vi "Gui_SetupTimingScript.vi"(7 "Variant For Path":variant, 8 "error in (no error)":errorcluster, 11 "Variant":variant) -> (0 "error out":errorcluster caption="sortie d'erreur", 3 "Variant Output":variant)   [LabVIEW 2018]
uses:
  controls/EXPERT_Inputs.ctl
  controls/DIGIT_5122_Inputs.ctl
  <instrlib>/niScope/Controls/niScope trigger source.ctl
  controls/HSDIO_6541_Inputs.ctl
  <instrlib>/niHSDIO/niHSDIO.llb/niHSDIO_ctl Trigger Source Values (Ring).ctl
  controls/SOFTWARE_Inputs.ctl
  controls/AO_6711_Inputs.ctl
  controls/AWG_5421_Inputs.ctl
  <instrlib>/niFgen/niFgen.llb/niFgen_ctl Trigger Source Values (Ring).ctl
  controls/XML_Inputs.ctl
  controls/SEQUENCE_Inputs.ctl
  controls/EXCIT_Inputs.ctl
  controls/DATA_Inputs.ctl
  controls/TIMING_Inputs.ctl
  controls/PROCESSING_Inputs.ctl
  controls/TRAPPING_Inputs.ctl
panel:
  in  "SEQUENCE Inputs":T1={"EXCIT Inputs"={"Number of Excitations"=1, "Script Text"="", "Table of Waveforms"=[]}, "DATA Inputs"={"Record Length"=524000, "Sample Rate"=2000000.0, "Data Type"=0, "Vertical Range"=10.0, "Acquisition Duration"=262.0}, "TIMING Inputs"={"Number of Acquisitions "=1, "Number of Accumulations"=1, "Table of Waveforms"=[], "Script Text"=""}, "PROCESSING Inputs"={"Reference Mass"=300.0939, "Cyclotron Freq"=255.727, "Magnetron Freq"=0.001}, "TRAPPING Inputs"={"Number of Channels"=4, "Init Values"=[2.0, 9.0, 2.0, 9.0], "Opening Values"=[0.0, 0.0, 0.0, 0.0], "Trapping Values"=[2.0, 9.0, 2.0, 9.0], "Emptying Values"=[-10.0, -10.0, -10.0, -10.0], "Adiabatic ON"=FALSE, "Adiabatic Duration"=100, "Adiabatic Waveforms"=["Adiabatic_None_2_2_2000", "Adiabatic_Ramp_9_0_2000", "Adiabatic_None_2_2_2000", "Adiabatic_RC_9_0_2000"], "Ions Refill ON"=FALSE, "Number of Ions Refills"=1, "Trapping Delay"=400.0, "Trapping Duration"=300.0}} {"TRAPPING Inputs"."Trapping Duration" min=2.0; "TRAPPING Inputs"."Trapping Delay" min=2.0; "TRAPPING Inputs"."Number of Ions Refills" min=1 max=1000; "TRAPPING Inputs"."Trapping Values" min=-10.0 max=10.0; "TRAPPING Inputs"."Init Values" min=-10.0 max=10.0; "TRAPPING Inputs"."Emptying Values" min=-10.0 max=10.0; "TRAPPING Inputs"."Opening Values" min=-10.0 max=10.0; "PROCESSING Inputs"."Magnetron Freq" format="%.5g"; "PROCESSING Inputs"."Cyclotron Freq" format="%.5g"; "PROCESSING Inputs"."Reference Mass" format="%.5g"; "TIMING Inputs"."Number of Accumulations" min=0 max=50 step=1; "TIMING Inputs"."Number of Acquisitions" min=1 max=10 step=1; "DATA Inputs"."Vertical Range" items=["0.2"=0.2, "0.4"=0.4, "1"=1.0, "2"=2.0, "4"=4.0, "10"=10.0]; "DATA Inputs"."Data Type" items=["I16", "DBL"]; "DATA Inputs"."Sample Rate" items=["1 MHz"=1000000.0, "2 MHz"=2000000.0, "5 MHz"=5000000.0, "10 MHz"=10000000.0, "20 MHz"=20000000.0, "25 MHz"=25000000.0, "50 MHz"=50000000.0, "100 MHz"=100000000.0]; "EXCIT Inputs"."Number of Excitations" min=1 max=10}
  out "Number Of Excitations":i16=1 min=1 max=10 step=1
  in  "Number Of Accumulations":i16=1 min=0 max=50 step=1
  out "Number Of Acquisitions":i16=1 min=1 max=10 step=1
  in  "OK":bool
  in  "CHECK":bool
  in  "EXPERT Inputs":T7={"DIGIT 5122 Inputs"={"Sample Rate"=10000.0, "Resource Name"="DIGIT_5122", "Channel Name"="0", "Trigger Source"="VAL_EXTERNAL", "Vertical Range"=10.0, "Trigger Level"=3.0}, "HSDIO 6541 Inputs"={"Resource Name"="HSDIO_6541", "Clock Rate"=1000000.0, "Trigger Source"="PFI0"}, "SOFTWARE Inputs"={"Application Directory"=path "D:/S.O.F.T.S/LABVIEW/PIL", "Software Version"="1.0.0", "Data Path"=path "D:/PIRENEA/DATA", "XML Path"=path "D:/PIRENEA/DATA", "XML File Filter"="*.xml", "XML Saved Path"=path "D:/PIRENEA/DATA/SAVED", "Excit Scripts Path"=path "D:/PIRENEA/EXCIT_SCRIPTS", "Excit Scripts File Filter"="*.txt", "Excit Waveforms Path"=path "D:/PIRENEA/EXCIT_WFMS", "Excit Waveforms File Filter"="*.bin", "Timing Scripts Path"=path "D:/PIRENEA/TECHNICAL/TIMING_SCRIPTS", "Timing Scripts File Filter"="*.txt", "Timing Waveforms Path"=path "D:/PIRENEA/TECHNICAL/TIMING_WFMS", "Timing Waveforms File Filter"="*.bin", "Trapping Waveforms Path"=path "D:/PIRENEA/TRAPPING_WFMS", "Trapping Waveforms File Filter"="*.bin"}, "AO 6711 Inputs"={"Physical Channels"="AO_6711/ao0:3", "Min Voltage"=-10.0, "Max Voltage"=10.0, "Trigger Source"="/AO_6711/PFI3", "Counter"="AO_6711/ctr0"}, "AWG 5421 Inputs"={"Resource Name"="AWG_5421", "Sample Rate"=10000000.0, "Trigger Type"=2, "Trigger Source"="PFI0", "Waveform Gain"=0.31, "Digital Filter ON"=TRUE}, "XML Inputs"={"Version Tag Name"="XML_Version", "Version String"="1.0"}} {"AWG 5421 Inputs"."Sample Rate" format="%.2p"; "AWG 5421 Inputs"."Trigger Type" items=["None", "Software Edge", "Digital Edge", "Digital Level"]; "AO 6711 Inputs"."Max Voltage" min=-10.0 max=10.0; "AO 6711 Inputs"."Min Voltage" min=-10.0 max=10.0; "HSDIO 6541 Inputs"."Clock Rate" format="%.2p"; "DIGIT 5122 Inputs"."Trigger Level" format="%.2f"; "DIGIT 5122 Inputs"."Vertical Range" format="%.2f"; "DIGIT 5122 Inputs"."Sample Rate" step=65535.0 format="%#_3p"}
  in  "Load":bool
  in  "Timing Script":string
  # "GO_out"
  # "Gout"
  # "GI_in"
  # "Gin"
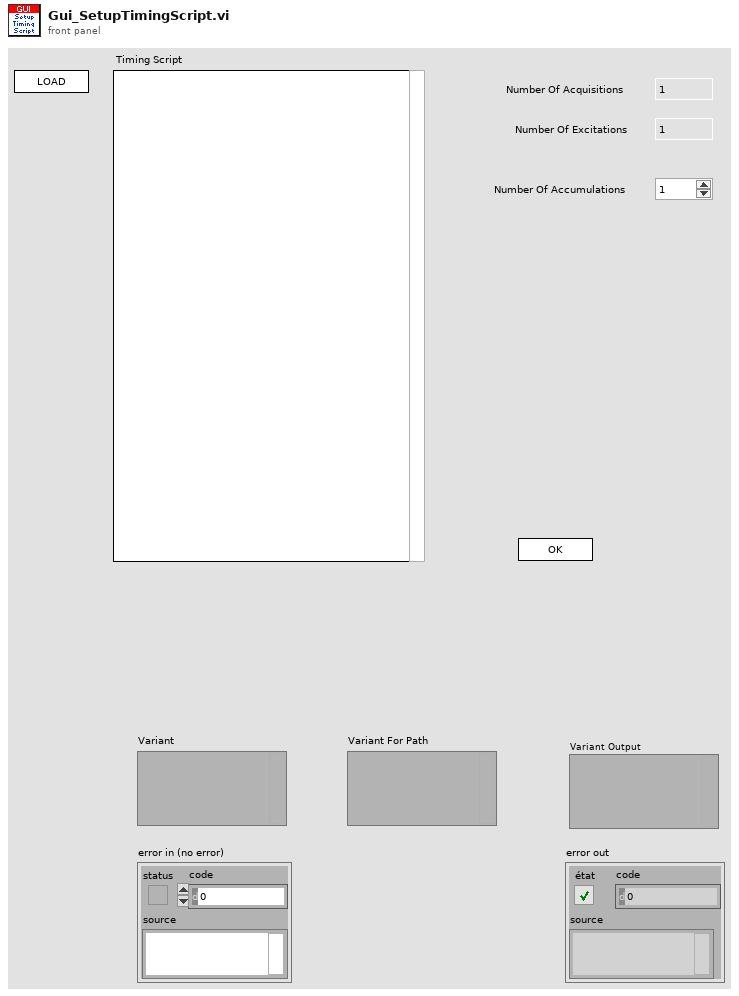
[diagram p1: front panel]
types:
  T1 = typedef "SEQUENCE_Inputs.ctl" = cluster{"EXCIT Inputs":T2, "DATA Inputs":T3, "TIMING Inputs":T4, "PROCESSING Inputs":T5, "TRAPPING Inputs":T6}
  T2 = typedef "EXCIT_Inputs.ctl" = cluster{"Number of Excitations":i32, "Script Text":string, "Table of Waveforms":string[]}
  T3 = typedef "DATA_Inputs.ctl" = cluster{"Record Length":i32, "Sample Rate":dbl, "Data Type":u8, "Vertical Range":dbl, "Acquisition Duration":dbl}
  T4 = typedef "TIMING_Inputs.ctl" = cluster{"Number of Acquisitions ":i16, "Number of Accumulations":i16, "Table of Waveforms":string[], "Script Text":string}
  T5 = typedef "PROCESSING_Inputs.ctl" = cluster{"Reference Mass":dbl, "Cyclotron Freq":dbl, "Magnetron Freq":dbl}
  T6 = typedef "TRAPPING_Inputs.ctl" = cluster{"Number of Channels":i32, "Init Values":dbl[], "Opening Values":dbl[], "Trapping Values":dbl[], "Emptying Values":dbl[], "Adiabatic ON":bool, "Adiabatic Duration":i32, "Adiabatic Waveforms":string[], "Ions Refill ON":bool, "Number of Ions Refills":i32, "Trapping Delay":dbl, "Trapping Duration":dbl}
  T7 = typedef "EXPERT_Inputs.ctl" = cluster{"DIGIT 5122 Inputs":T8, "HSDIO 6541 Inputs":T10, "SOFTWARE Inputs":T12, "AO 6711 Inputs":T13, "AWG 5421 Inputs":T14, "XML Inputs":T16}
  T8 = typedef "DIGIT_5122_Inputs.ctl" = cluster{"Sample Rate":dbl, "Resource Name":refnum<k15>, "Channel Name":string, "Trigger Source":T9, "Vertical Range":dbl, "Trigger Level":dbl}
  T9 = typedef "niScope trigger source.ctl" = string
  T10 = typedef "HSDIO_6541_Inputs.ctl" = cluster{"Resource Name":refnum<k15>, "Clock Rate":dbl, "Trigger Source":T11}
  T11 = typedef "niHSDIO_ctl Trigger Source Values (Ring).ctl" = string
  T12 = typedef "SOFTWARE_Inputs.ctl" = cluster{"Application Directory":path, "Software Version":string, "Data Path":path, "XML Path":path, "XML File Filter":string, "XML Saved Path":path, "Excit Scripts Path":path, "Excit Scripts File Filter":string, "Excit Waveforms Path":path, "Excit Waveforms File Filter":string, "Timing Scripts Path":path, "Timing Scripts File Filter":string, "Timing Waveforms Path":path, "Timing Waveforms File Filter":string, "Trapping Waveforms Path":path, "Trapping Waveforms File Filter":string}
  T13 = typedef "AO_6711_Inputs.ctl" = cluster{"Physical Channels":tag, "Min Voltage":dbl, "Max Voltage":dbl, "Trigger Source":tag, "Counter":tag}
  T14 = typedef "AWG_5421_Inputs.ctl" = cluster{"Resource Name":refnum<k15>, "Sample Rate":dbl, "Trigger Type":u16, "Trigger Source":T15, "Waveform Gain":dbl, "Digital Filter ON":bool}
  T15 = typedef "niFgen_ctl Trigger Source Values (Ring).ctl" = string
  T16 = typedef "XML_Inputs.ctl" = cluster{"Version Tag Name":string, "Version String":string}
  T17 = enum16{"Native", "Native Command Line", "UNIX", "Macintosh", "DOS"}
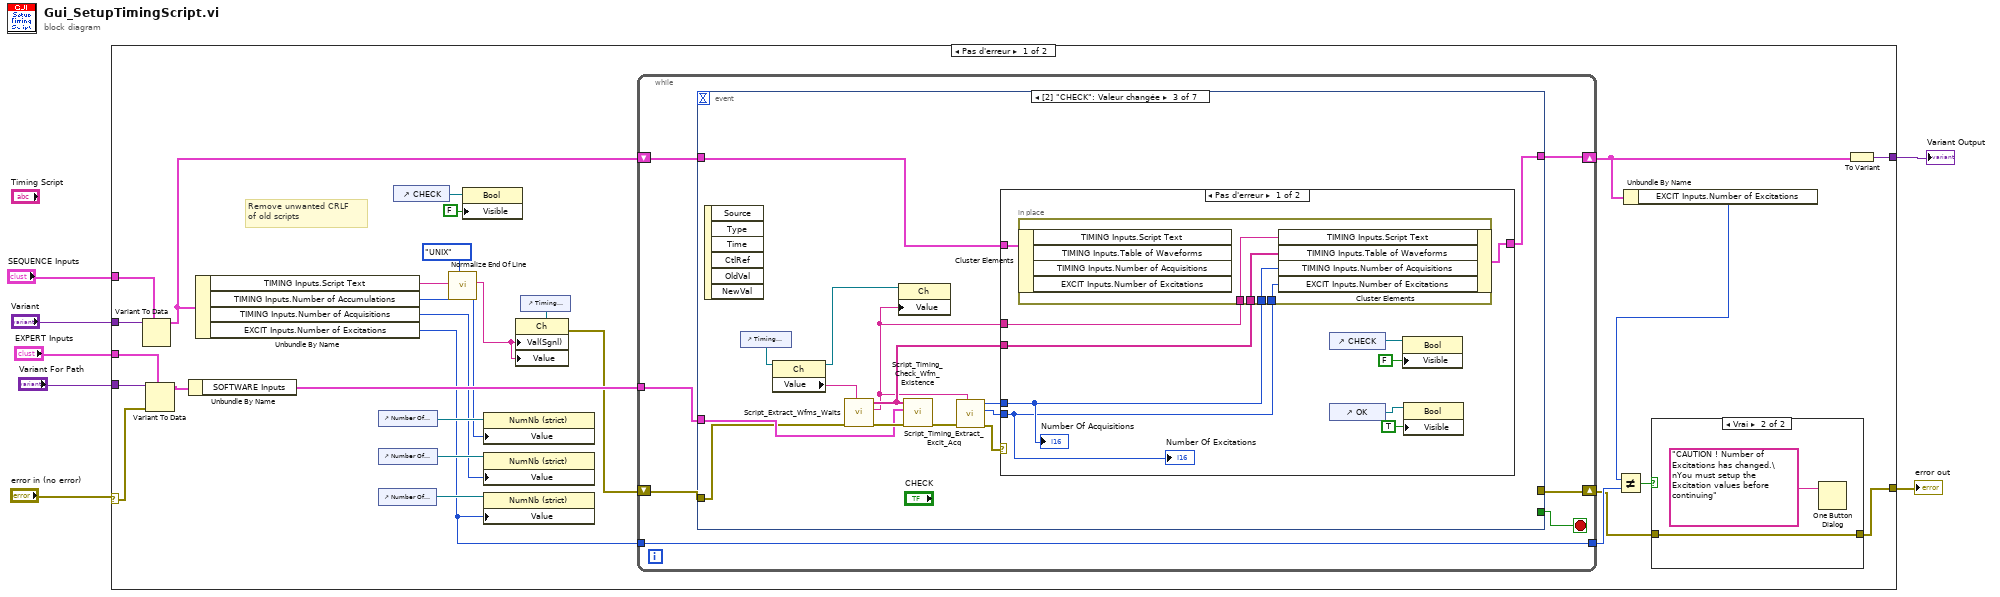
[diagram p0: block diagram]
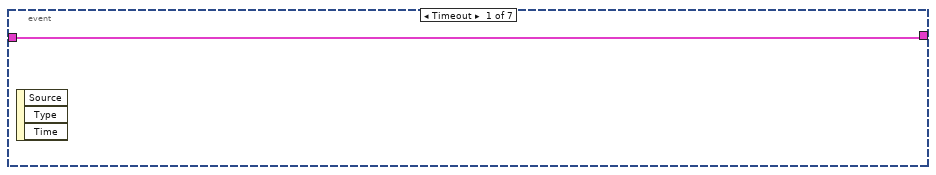
[diagram p3: hidden frame]
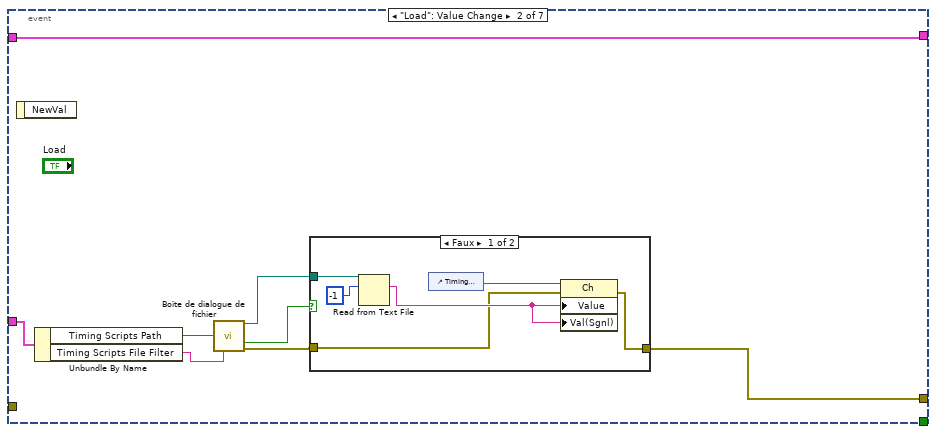
[diagram p4: hidden frame]
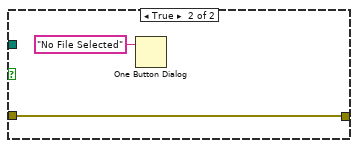
[diagram p5: hidden frame]
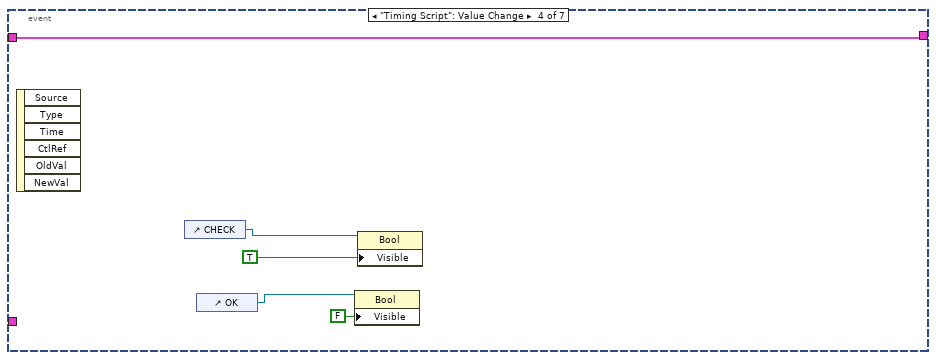
[diagram p7: hidden frame]
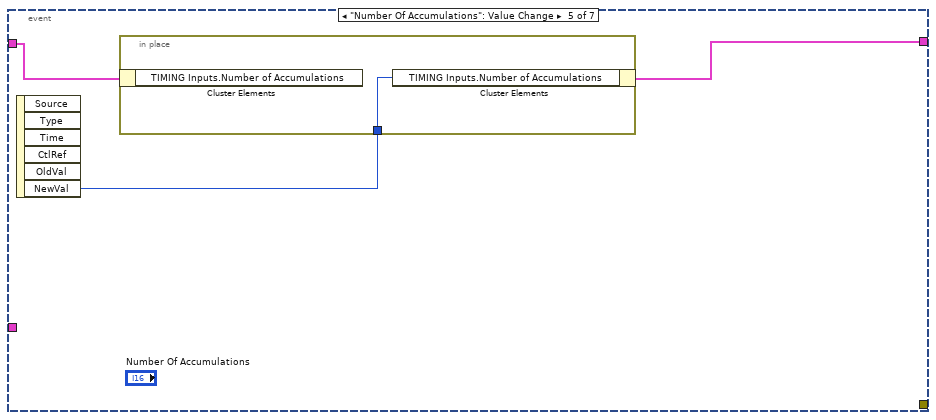
[diagram p8: hidden frame]
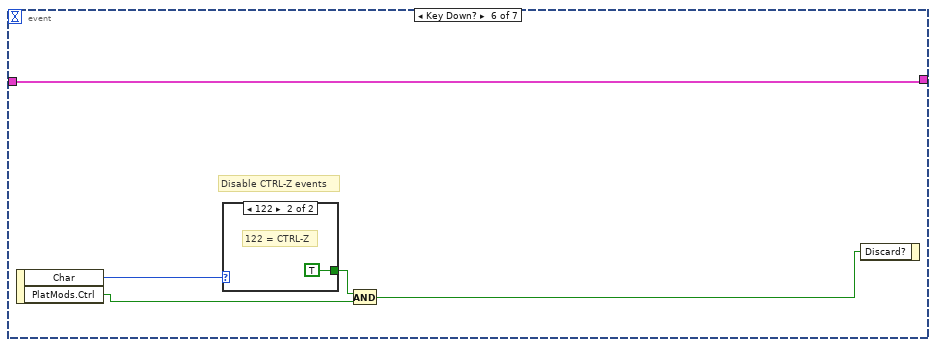
[diagram p9: hidden frame]
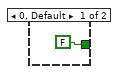
[diagram p10: hidden frame]
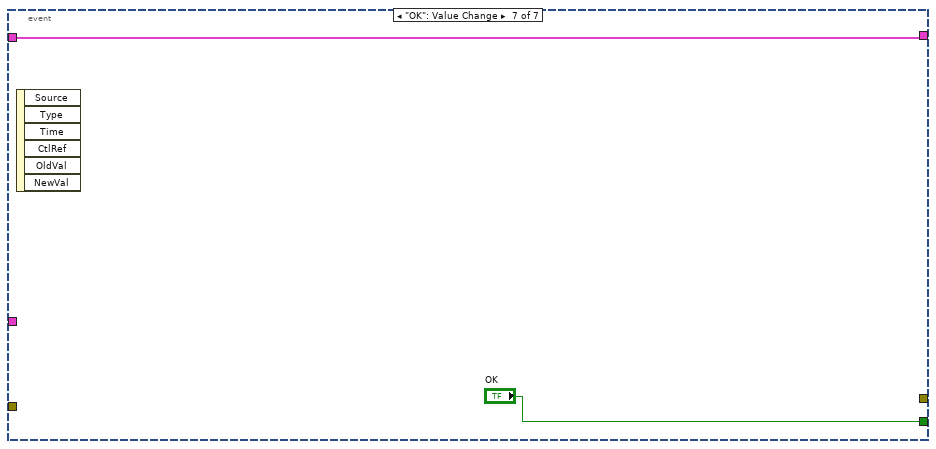
[diagram p11: hidden frame]
diagram:
  n1 = case shown="Pas d'erreur" "error in (no error)" {
    selector: "error in (no error)" -> [w29 w110]
    tunnel: "Variant" -> [w35 _]
    tunnel: [w13 w110] -> w5
    tunnel: "SEQUENCE Inputs" -> [w21 _]
    tunnel: "EXPERT Inputs" -> [w22 _]
    tunnel: "Variant For Path" -> [w30 _]
    tunnel: [w20 _] -> w2
    frame No Error {
      # "Remove unwanted CRLF\nof old scripts"
      n2 = Variant To Data(type=w21, Variant=w35) -> (data=w18:T1)  [unwired: 1 in, 1 out]
      n3 = Variant To Data(error in=w29, type=w22, Variant=w30) -> (data=w19:T7)  [unwired: 1 out]
      n4 = Unbundle By Name(w19) -> ("SOFTWARE Inputs"=w33:T12)
      n5 = Unbundle By Name(w18) -> ("TIMING Inputs.Script Text"=w10:string, "TIMING Inputs.Number of Accumulations"=w26:i16, "TIMING Inputs.Number of Acquisitions"=w24:i16, "EXCIT Inputs.Number of Excitations"=w17:i32)
      n6 = control-ref of="Number Of Excitations"() -> (w23:refnum<vi>)
      n7 = control-ref of="Number Of Accumulations"() -> (w27:refnum<vi>)
      n8 = control-ref of="Number Of Acquisitions"() -> (w25:refnum<vi>)
      n9 = control-ref of="CHECK"() -> (w31:refnum<vi>)
      n10 = call <vilib>:"Normalize End Of Line.vi"("end of line (Native)"=T17."UNIX", "string in"=w10) -> ("string out"=w8:string)  [unwired: 6 in]
      n11 = property class="Bool"(reference=w31, "Visible"=FALSE) -> ()  [unwired: 1 in, 2 out]
      n12 = property class="NumNb (strict)"(reference=w27, "Value"=w26) -> ()  [unwired: 1 in, 2 out]
      n13 = property class="NumNb (strict)"(reference=w25, "Value"=w24) -> ()  [unwired: 1 in, 2 out]
      n14 = property class="NumNb (strict)"(reference=w23, "Value"=w17) -> ()  [unwired: 1 in, 2 out]
      n15 = control-ref of="Timing Script"() -> (w34:refnum<vi>)
      n16 = property class="Ch"(reference=w34, "Val(Sgnl)"=w8, "Value"=w8) -> (error out=w28:errorcluster)  [unwired: 1 in, 1 out]
      n17 = while {
        shift-right: [w43] -> w14
        shift-left: w28 -> [w45]
        tunnel: w33 -> [w40]
        shift-right: [w41] -> w12
        shift-left: w18 -> [w42]
        tunnel: w17 -> [w39]
        tunnel: [w39] -> w15
        stop <- w44 stop-if-true
        n18 = event shown="[2] \"CHECK\": Valeur changée" {
          selector: _ -> [_ _ _ _ _ _ _]
          dyn-events: _ -> [_ _ _ _ _ _ _]
          timeout: _ -> [_ _ _ _ _ _ _]
          tunnel: w45 -> [_ _ w63 _ _ _ _]
          tunnel: [_ w50 _ _ _ _ _] -> w43
          tunnel: [_ _ _ _ _ _ "OK"] -> w44
          tunnel: w42 -> [w46 w51 w74 w94 w99 w101 w108]
          tunnel: [w46 w51 w73 w94 w97 w101 w108] -> w41
          tunnel: w40 -> [_ w49 w71 _ _ _ _]
          event Timeout {
            n19 = event-data() -> ()  [unwired: 1 in, 3 out]
          }
          event "Load": Value Change {
            n20 = event-data() -> ()  [unwired: 1 in, 1 out]
            n21 = Unbundle By Name(w49) -> ("Timing Scripts Path"=w47:path, "Timing Scripts File Filter"=w48:string)
            n22 = call "Boîte de dialogue de fichier"("start path"=w47, "pattern (all files)"=w48) -> ("selected path"=w54:path, "cancelled"=w53:bool, "error out"=w52:errorcluster)  [unwired: 10 in, 1 out]
            n23 = case shown="Faux" w53 {
              tunnel: w54 -> [w60 _]
              tunnel: w52 -> [w56 w61]
              tunnel: [w55 w61] -> w50
              frame False {
                n24 = Read from Text File(file (use dialog)=w60, count=-1 ("nombre")) -> (text=w57:string)  [unwired: 2 in, 3 out]
                n25 = control-ref of="Timing Script"() -> (w58:refnum<vi>)
                n26 = property class="Ch"(reference=w58, error in=w56, "Value"=w57, "Val(Sgnl)"=w57) -> (error out=w55:errorcluster)  [unwired: 1 out]
              }
              frame True {
                n27 = One Button Dialog(message="No File Selected") -> ()  [unwired: 1 in, 1 out]
              }
            }
          }
          event "CHECK": Value Change {
            n28 = event-data() -> ()  [unwired: 1 in, 6 out]
            n29 = control-ref of="Timing Script"() -> (w76:refnum<vi>)
            n30 = property class="Ch"(reference=w76) -> (reference out=w64:refnum<vi>, "Value"=w68:string)  [unwired: 1 in, 1 out]
            n31 = call "Script_Extract_Wfms_Waits.vi"("Script Text"=w68, "error in (no error)"=w63) -> ("error out"=w75:errorcluster, "Script Text Cleaned"=w65:string, "Table of Loaded Wfms"=w72:string[])  [unwired: 6 in, 1 out]
            n32 = property class="Ch"(reference=w64, "Value"=w65) -> ()  [unwired: 1 in, 2 out]
            n33 = call "Script_Timing_Check_Wfm_Existence.vi"("error  in"=w75, "SOFTWARE Inputs"=w71, "Table of Waveforms"=w72) -> ("error out"=w70:errorcluster)  [unwired: 8 in]
            n34 = call "Script_Timing_Extract_Excit_Acq.vi"("Script Text"=w65, "error in (no error)"=w70) -> ("error out"=w69:errorcluster, "Number of Excits"=w66:i16, "Number of Acqs"=w67:i16)  [unwired: 7 in]
            n35 = case shown="Pas d'erreur" w69 {
              tunnel: w74 -> [w84 w91]
              tunnel: [w83 w91] -> w73
              tunnel: w65 -> [w82 _]
              tunnel: w72 -> [w81 _]
              tunnel: w67 -> [w80 _]
              tunnel: w66 -> [w79 _]
              frame No Error {
                n36 = in-place {
                  in-place-border: w82 -> [w90]
                  in-place-border: w81 -> [w89]
                  in-place-border: w80 -> [w88]
                  in-place-border: w79 -> [w87]
                  n37 = in-place-cluster #1(w84) -> ()  [unwired: 4 out]
                  n38 = in-place-cluster #1("TIMING Inputs.Script Text"=w90, "TIMING Inputs.Table of Waveforms"=w89, "TIMING Inputs.Number of Acquisitions"=w88, "EXCIT Inputs.Number of Excitations"=w87) -> (w83:T1)
                }
                n39 = control-ref of="CHECK"() -> (w86:refnum<vi>)
                n40 = control-ref of="OK"() -> (w78:refnum<vi>)
                n41 = property class="Bool"(reference=w86, "Visible"=FALSE) -> ()  [unwired: 1 in, 2 out]
                n42 = property class="Bool"(reference=w78, "Visible"=TRUE) -> ()  [unwired: 1 in, 2 out]
                "Number Of Acquisitions" <- w80
                "Number Of Excitations" <- w79
              }
              frame Error {
              }
            }
          }
          event "Timing Script": Value Change {
            n43 = event-data() -> ()  [unwired: 1 in, 6 out]
            n44 = control-ref of="CHECK"() -> (w96:refnum<vi>)
            n45 = control-ref of="OK"() -> (w93:refnum<vi>)
            n46 = property class="Bool"(reference=w93, "Visible"=FALSE) -> ()  [unwired: 1 in, 2 out]
            n47 = property class="Bool"(reference=w96, "Visible"=TRUE) -> ()  [unwired: 1 in, 2 out]
          }
          event "Number Of Accumulations": Value Change {
            n48 = event-data() -> ("NewVal"=w98:i16)  [unwired: 1 in, 5 out]
            n49 = in-place {
              in-place-border: w98 -> [w100]
              n50 = in-place-cluster #2(w99) -> ()  [unwired: 1 out]
              n51 = in-place-cluster #2("TIMING Inputs.Number of Accumulations"=w100) -> (w97:T1)
            }
          }
          event Key Down? {
            # "Disable CTRL-Z events"
            n52 = event-data() -> ("Char"=w104:i16, "PlatMods.Ctrl"=w103:bool)  [unwired: 1 in]
            n53 = case shown="122" w104 {
              tunnel: [FALSE TRUE] -> w105
              frame 0, Default {
              }
              frame 122 {
                # "122 = CTRL-Z"
              }
            }
            n54 = And(x=w105, y=w103) -> (x .and. y?=w102:bool)
            n55 = event-data("Discard?"=w102) -> ()  [unwired: 1 in, 1 out]
          }
          event "OK": Value Change {
            n56 = event-data() -> ()  [unwired: 1 in, 6 out]
          }
        }
      }
      n57 = Unbundle By Name(w12) -> ("EXCIT Inputs.Number of Excitations"=w11:i32)
      n58 = Not Equal?(x=w11, y=w15) -> (x != y?=w16:bool)
      n59 = case shown="Vrai" w16 {
        tunnel: w14 -> [w36 w37]
        tunnel: [w36 w37] -> w13
        frame False {
        }
        frame True {
          n60 = One Button Dialog(message="CAUTION ! Number of Excitations has changed.\nYou must setup the Excitation values before continuing") -> ()  [unwired: 1 in, 1 out]
        }
      }
      n61 = To Variant(anything=w12) -> (Variant=w20:variant)
    }
    frame Error {
    }
  }
  "error out" <- w5
  "Variant Output" <- w2
